vi "Launch Vacuum.vi"(8 "error in (no error)":errorcluster, 11 "cRIO-CO2 in":refnum<class "cRIO-CO2.lvclass">) -> (0 "error out":errorcluster, 3 "cRIO-CO2 out":refnum<class "cRIO-CO2.lvclass">)   [LabVIEW 2015, in "cRIO-Carbondioxide.lvlib" / "cRIO-CO2.lvlib" / "cRIO-CO2.lvclass"]
uses:
  cRIO-CO2.lvclass
  cRIO-CO2.lvclass/cRIO-CO2.ctl
  CO2 Actor Messages/Ping Msg/Ping Msg.lvclass/Ping Msg.ctl
  <vilib>/ActorFramework/Message Enqueuer/Message Enqueuer.lvclass/Message Enqueuer.ctl
  <vilib>/ActorFramework/Actor/Actor.lvclass
  <vilib>/ActorFramework/Message Enqueuer/Enqueue.vi
  <vilib>/ActorFramework/Message Priority Queue/Priority Enqueue.vi
  CO2 Actor Messages/Ping Msg/Ping Msg.lvclass
  <vilib>/ActorFramework/Message Enqueuer/Message Enqueuer.lvclass
  cRIO Vacuum/cRIO Vacuum.lvclass
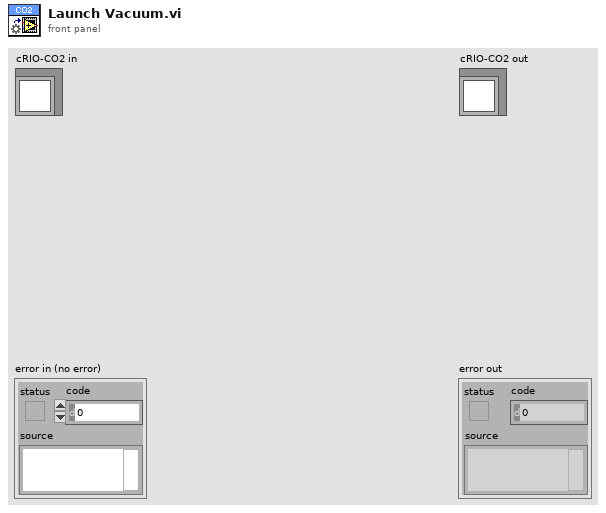
[diagram p1: front panel]
types:
  T1 = typedef "Dedicated Enqueuers.ctl" = cluster{"Freezers":cluster{"Syringe":refnum<class "Message Enqueuer.lvclass">, "Tank 1":refnum<class "Message Enqueuer.lvclass">, "Tank 2":refnum<class "Message Enqueuer.lvclass">, "Tank 3":refnum<class "Message Enqueuer.lvclass">, "Tank 4":refnum<class "Message Enqueuer.lvclass">}, "Heaters":cluster{"Syringe":refnum<class "Message Enqueuer.lvclass">, "Piston":refnum<class "Message Enqueuer.lvclass">}, "Blowers":cluster{"Tank 1":refnum<class "Message Enqueuer.lvclass">, "Tank 2":refnum<class "Message Enqueuer.lvclass">, "Tank 3":refnum<class "Message Enqueuer.lvclass">, "Tank 4":refnum<class "Message Enqueuer.lvclass">, "Syringe":refnum<class "Message Enqueuer.lvclass">}, "Sample Line":refnum<class "Message Enqueuer.lvclass">, "Storage Line":refnum<class "Message Enqueuer.lvclass">, "Transfer Line":refnum<class "Message Enqueuer.lvclass">, "Syringe Stepper":refnum<class "Message Enqueuer.lvclass">, "Syringe Line":refnum<class "Message Enqueuer.lvclass">, "Capillary Line":refnum<class "Message Enqueuer.lvclass">, "Preparation Line":refnum<class "Message Enqueuer.lvclass">, "Turbo":refnum<class "Message Enqueuer.lvclass">, "Vacuum":refnum<class "Message Enqueuer.lvclass">, "He Line":refnum<class "Message Enqueuer.lvclass">, "Cylinder":refnum<class "Message Enqueuer.lvclass">}
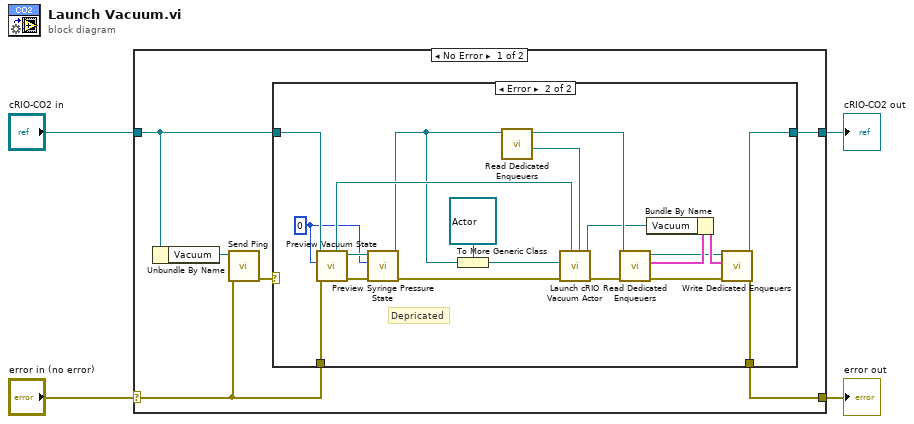
[diagram p0: block diagram]
diagram:
  n1 = case shown="No Error" "error in (no error)" {
    selector: "error in (no error)" -> [w5 w34]
    tunnel: [w9 w34] -> w3
    tunnel: "cRIO-CO2 in" -> [w8 w33]
    tunnel: [w10 w33] -> w1
    frame No Error {
      n2 = Unbundle By Name(w8) -> ("Vacuum"=w7:refnum<class "Message Enqueuer.lvclass">)
      n3 = call "Send Ping.vi"("error in (no error)"=w5, "Message Enqueuer"=w7) -> ("error out"=w6:errorcluster)  [unwired: 6 in, 3 out]
      n4 = case shown="Error" w6 {
        tunnel: [w11 w25] -> w10
        tunnel: [w12 w21] -> w9
        tunnel: w8 -> [w11 w20]
        tunnel: w5 -> [w12 w19]
        frame No Error {
        }
        frame Error {
          w13 = 0 ("timeout in ms (-1)")
          # "Depricated"
          n5 = call "Preview Vacuum State.vi"("error in (no error)"=w19, "timeout in ms (-1)"=w13, "cRIO-CO2 in"=w20) -> ("error out"=w17:errorcluster, "cRIO-CO2 out"=w15:refnum<class "cRIO-CO2.lvclass">, "Vacuum StateQ"=w18:refnum<queue>)  [unwired: 2 in, 4 out]
          n6 = call "Preview Syringe Pressure State.vi"("error in (no error)"=w17, "timeout in ms (-1)"=w13, "cRIO-CO2 in"=w15) -> ("error out"=w16:errorcluster, "cRIO-CO2 out"=w14:refnum<class "cRIO-CO2.lvclass">)  [unwired: 2 in, 5 out]
          n7 = To More Generic Class(target class=refnum<class "Actor.lvclass"> refnum ("Caller Actor in"), reference=w14) -> (generic class reference=w23:refnum<class "Actor.lvclass">)
          n8 = call "Read Dedicated Enqueuers.vi"("cRIO-CO2 in"=w14) -> ("Qs.DedicatedEnQrs"=w28:refnum<queue>, "cRIO-CO2 out"=w26:refnum<class "cRIO-CO2.lvclass">)  [unwired: 7 in, 2 out]
          n9 = call "Launch cRIO Vacuum Actor.vi"("DedicatedEnQrs"=w28, "Vacuum StateQ"=w18, "error in (no error)"=w16, "Caller Actor in"=w23) -> ("error out"=w27:errorcluster, "Caller-To-Actor Enqueuer"=w24:refnum<class "Message Enqueuer.lvclass">)  [unwired: 6 in]
          n10 = call "Read Dedicated Enqueuers.vi"("error in (no error)"=w27, "cRIO-CO2 in"=w26) -> ("error out"=w29:errorcluster, "Dedicated Enqueuers"=w31:T1, "cRIO-CO2 out"=w30:refnum<class "cRIO-CO2.lvclass">)  [unwired: 6 in, 1 out]
          n11 = Bundle By Name(cluster=w31, "Vacuum"=w24) -> (w32:T1)
          n12 = call "Write Dedicated Enqueuers.vi"("error in (no error)"=w29, "Dedicated Enqueuers"=w32, "cRIO-CO2 in"=w30) -> ("error out"=w21:errorcluster, "cRIO-CO2 out"=w25:refnum<class "cRIO-CO2.lvclass">)  [unwired: 7 in]
        }
      }
    }
    frame Error {
    }
  }
  "error out" <- w3
  "cRIO-CO2 out" <- w1
